vi "DeviceReplyTo.vi"(11 "Device":string) -> (2 "ReplyTo":string)   [LabVIEW 2017]
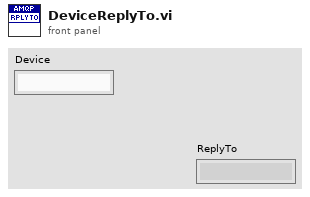
[diagram p1: front panel]
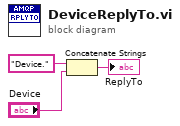
[diagram p0: block diagram]
diagram:
  n1 = Concatenate Strings("Device." ("string"), "Device") -> (→"ReplyTo":string)
